vi "RSZVB Delete Port Pair.vi"(7 "Port Pair (1)":i32=1, 8 "error in (no error)":errorcluster {"code" format="%.0x"}, 9 "Function Type (Deembedding)":i32(ring) items=["Deembedding", "Embedding"], 10 "Channel (1)":i32=1, 11 "VISA session":refnum<visa-resource-name>) -> (0 "error out":errorcluster {"code" format="%.0x"}, 3 "dup VISA session":refnum<visa-resource-name>)   [LabVIEW 2011]
doc: "Deletes the previously defined list of port pairs for port pair embedding/deembedding.\n\nRemote-control command(s):\nCALCulate<Ch>:TRANsform:VNETworks:PPAir:DEEMbedding<List_idx>:DELete\nCALCulate<Ch>:TRANsform:VNETworks:PPAir:EMBedding<List_idx>:DELete"
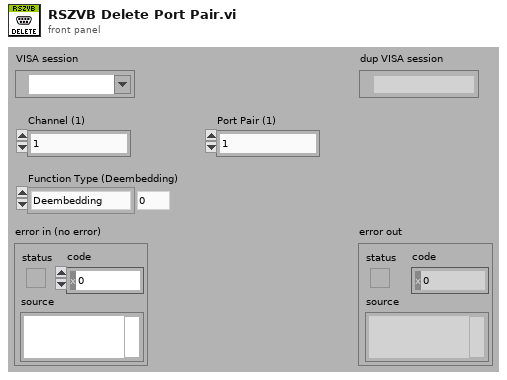
[diagram p1: front panel]
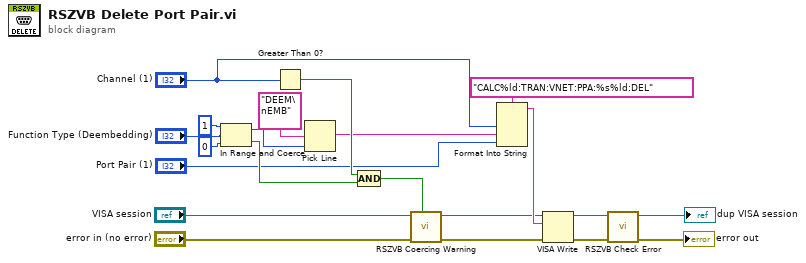
[diagram p0: block diagram]
diagram:
  n1 = In Range and Coerce(upper limit=1, x="Function Type (Deembedding)", lower limit=0) -> (coerced(x)=w8:i32, In Range?=w7:bool)
  n2 = Greater Than 0?(x="Channel (1)") -> (x > 0?=w17:bool)
  n3 = Pick Line(multi-line string="DEEM\nEMB", line index=w8) -> (output string=w9:string)  [unwired: 1 in]
  n4 = Compound Arithmetic op=AND(w17, w7) -> (w16:bool)
  n5 = call "RSZVB Coercing Warning.vi"("In Range?"=w16, "error in (no error)"="error in (no error)", "VISA session"="VISA session") -> ("error out"=w20:errorcluster, "dup VISA session"=w19:refnum<visa-resource-name>)  [unwired: 7 in]
  n6 = Format Into String(format string="CALC%ld:TRAN:VNET:PPA:%s%ld:DEL", "Channel (1)", w9, "Port Pair (1)") -> (resulting string=w21:string)  [unwired: 2 in, 1 out]
  n7 = VISA Write(VISA resource name=w19, write buffer=w21, error in (no error)=w20) -> (VISA resource name out=w15:refnum<visa-resource-name>, error out=w14:errorcluster)  [unwired: 1 out]
  n8 = call "RSZVB Check Error.vi"("error in (no error)"=w14, "VISA session"=w15) -> ("error out"=→"error out":errorcluster, "dup VISA session"=→"dup VISA session":refnum<visa-resource-name>)  [unwired: 8 in]
